vi "Calibration_Load.vi"(11 "Data in":T2={"system"={"info"={"menuSelect"=0, "version"=0, "serial"="Test Sample", "captureActive"=FALSE, "captureBegin"=FALSE, "emptyAndRefill"=FALSE}, "userInfo"={"operatorName"="", "date"=timestamp(2713993200 s since 1904-01-01)}, "camera"={"exposureTime"=0, "aperture"=enum."Item 0", "framerate"=0, "framerateMax"=500, "legacyAttributes"=FALSE}}, "connections"={"arduino"={"connection"="", "status"=FALSE, "openState"=FALSE, "emptyStart"=0}, "pump"={"connection"="MRJ", "status"=FALSE, "command"="", "dispenseSpeed"=100, "flushSize"=100}, "camera"={"cam1"={"connection"="", "status"=FALSE}, "cam2"={"connection"="", "status"=FALSE}}}, "queue"={"process"={"cam1"=refnum, "cam2"=refnum, "queueSize"=0}, "save"={"cam1"=refnum, "cam2"=refnum, "queueSize"=0}, "overloadThreshold"=0}, "imageProcess"={"cam1"={"preAllocation"={"image"="Station", "originalDisplay"="Station", "originalRgb"="Station", "binary"="Station", "save"="Station", "calibrationFull"=refnum, "calibrationDetect"=refnum}, "calibration"={"pathFull"=path "C:/Users/au540322/Desktop/IHS_Project/images/Debris/Debris_0/Debris_0_2019_06_01-23-32-49-686.PNG", "pathDetect"=path "C:/Users/au540322/Desktop/IHS_Project/images/Debris/Debris_0/Debris_0_2019_06_01-23-32-49-686.PNG", "ROI"={"Left"=0, "Top"=0, "Right"=0, "Bottom"=0, "Rotation"=0.0}}}, "cam2"={"preAllocation"={"image"=refnum, "originalDisplay"=refnum, "originalRgb"=refnum, "binary"=refnum, "save"=refnum, "calibrationFull"=refnum, "calibrationDetect"=refnum}, "calibration"={"pathFull"=path "C:/Users/au540322/Desktop/IHS_Project/images/Debris/Debris_0/Debris_0_2019_06_01-23-32-49-686.PNG", "pathDetect"=path "C:/Users/au540322/Desktop/IHS_Project/images/Debris/Debris_0/Debris_0_2019_06_01-23-32-49-686.PNG", "ROI"={"Left"=0, "Top"=0, "Right"=0, "Bottom"=0, "Rotation"=0.0}}}, "process"={"planeExtract"=refnum, "planeSubtract"=refnum, "cropMask"=refnum}, "detection"={"sampleTimeout"=500, "sizeThreshold"=500, "detectionRegionPct"=0.0}}, "sampleData"={"sampleId"="", "projectId"="", "voucherID"="", "speciesName"="", "collectionDate"=timestamp(2713993200 s since 1904-01-01), "sampleStation"="", "location"="", "lat"=0.0, "lon"=0.0, "determiner"="", "sex"="", "otherNotes"=""}, "Session In"=""} {"sampleData"."collectionDate" format="%<%Y-%m-%d>T"; "imageProcess"."detection"."sizeThreshold" min=1; "imageProcess"."cam2"."calibration"."ROI"."Rotation" format="%.2f"; "imageProcess"."cam2"."calibration"."ROI"."Left" scale=0.0..1024.0; "imageProcess"."cam2"."calibration"."ROI"."Right" scale=0.0..1024.0; "imageProcess"."cam1"."calibration"."ROI"."Rotation" format="%.2f"; "imageProcess"."cam1"."calibration"."ROI"."Left" scale=0.0..1024.0; "imageProcess"."cam1"."calibration"."ROI"."Right" scale=0.0..1024.0; "queue"."overloadThreshold" min=1; "queue"."save"."queueSize" min=1; "queue"."process"."queueSize" min=1; "connections"."pump"."flushSize" min=1; "connections"."pump"."dispenseSpeed" min=1; "system"."camera"."framerateMax" min=1; "system"."userInfo"."date" format="%<%Y-%m-%dT%H:%M:%S+%z>T"; "system"."info"."version" items=["Standard", "XL"]; "system"."info"."menuSelect" items=["Session Data", "Extended Setup", "Buffer", "Camera", "Dispenser", "Stats", "Connections"]}) -> (0 "Next State":T1=enum."Wait for Event", 2 "Calibration error?":bool, 3 "Data out":T2={"system"={"info"={"menuSelect"=0, "version"=0, "serial"="Test Sample", "captureActive"=FALSE, "captureBegin"=FALSE, "emptyAndRefill"=FALSE}, "userInfo"={"operatorName"="", "date"=timestamp(2713993200 s since 1904-01-01)}, "camera"={"exposureTime"=0, "aperture"=enum."Item 0", "framerate"=0, "framerateMax"=500, "legacyAttributes"=FALSE}}, "connections"={"arduino"={"connection"="", "status"=FALSE, "openState"=FALSE, "emptyStart"=0}, "pump"={"connection"="", "status"=FALSE, "command"="", "dispenseSpeed"=100, "flushSize"=100}, "camera"={"cam1"={"connection"="", "status"=FALSE}, "cam2"={"connection"="", "status"=FALSE}}}, "queue"={"process"={"cam1"=refnum, "cam2"=refnum, "queueSize"=0}, "save"={"cam1"=refnum, "cam2"=refnum, "queueSize"=0}, "overloadThreshold"=0}, "imageProcess"={"cam1"={"preAllocation"={"image"="Station", "originalDisplay"="Station", "originalRgb"="Station", "binary"="Station", "save"="Station", "calibrationFull"=refnum, "calibrationDetect"=refnum}, "calibration"={"pathFull"=path "C:/Users/au540322/Desktop/IHS_Project/images/Debris/Debris_0/Debris_0_2019_06_01-23-32-49-686.PNG", "pathDetect"=path "C:/Users/au540322/Desktop/IHS_Project/images/Debris/Debris_0/Debris_0_2019_06_01-23-32-49-686.PNG", "ROI"={"Left"=0, "Top"=0, "Right"=0, "Bottom"=0, "Rotation"=0.0}}}, "cam2"={"preAllocation"={"image"=refnum, "originalDisplay"=refnum, "originalRgb"=refnum, "binary"=refnum, "save"=refnum, "calibrationFull"=refnum, "calibrationDetect"=refnum}, "calibration"={"pathFull"=path "C:/Users/au540322/Desktop/IHS_Project/images/Debris/Debris_0/Debris_0_2019_06_01-23-32-49-686.PNG", "pathDetect"=path "C:/Users/au540322/Desktop/IHS_Project/images/Debris/Debris_0/Debris_0_2019_06_01-23-32-49-686.PNG", "ROI"={"Left"=0, "Top"=0, "Right"=0, "Bottom"=0, "Rotation"=0.0}}}, "process"={"planeExtract"=refnum, "planeSubtract"=refnum, "cropMask"=refnum}, "detection"={"sampleTimeout"=500, "sizeThreshold"=500, "detectionRegionPct"=0.0}}, "sampleData"={"sampleId"="", "projectId"="", "voucherID"="", "speciesName"="", "collectionDate"=timestamp(2713993200 s since 1904-01-01), "sampleStation"="", "location"="", "lat"=0.0, "lon"=0.0, "determiner"="", "sex"="", "otherNotes"=""}, "Session In"=""} {"sampleData"."collectionDate" format="%<%Y-%m-%d>T"; "imageProcess"."detection"."sizeThreshold" min=1; "imageProcess"."cam2"."calibration"."ROI"."Rotation" format="%.2f"; "imageProcess"."cam2"."calibration"."ROI"."Left" scale=0.0..1024.0; "imageProcess"."cam2"."calibration"."ROI"."Right" scale=0.0..1024.0; "imageProcess"."cam1"."calibration"."ROI"."Rotation" format="%.2f"; "imageProcess"."cam1"."calibration"."ROI"."Left" scale=0.0..1024.0; "imageProcess"."cam1"."calibration"."ROI"."Right" scale=0.0..1024.0; "queue"."overloadThreshold" min=1; "queue"."save"."queueSize" min=1; "queue"."process"."queueSize" min=1; "connections"."pump"."flushSize" min=1; "connections"."pump"."dispenseSpeed" min=1; "system"."camera"."framerateMax" min=1; "system"."userInfo"."date" format="%<%Y-%m-%dT%H:%M:%S+%z>T"; "system"."info"."version" items=["Standard", "XL"]; "system"."info"."menuSelect" items=["Session Data", "Extended Setup", "Buffer", "Camera", "Dispenser", "Stats", "Connections"]})   [LabVIEW 2022 SP3]
uses:
  controls/Data.ctl
  <vilib>/userdefined/High Color/IMAQdx.ctl
  <vilib>/vision/Image Controls.llb/IMAQ Image.ctl
  controls/State.ctl
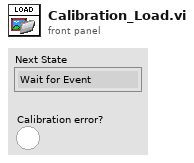
[diagram p1: front panel]
types:
  T1 = typedef "State.ctl" = enum16{"Initialize", "Wait for Event", "Position", "Valve Signal", "Extra Flush", "Valve Cycle", "Valve Open", "Valve Close", "Pump Command", "Pump Cycle", "Empty System", "Start System", "Connect Systems", "Start Image Capture", "Stop Image Capture", "Calibration Pictures", "Close and Refill", "Empty and Refill", "Change Light Intensity", "Reconnect", "CursorIdle", "Exit"}
  T2 = typedef "Data.ctl" = cluster{"system":cluster{"info":cluster{"menuSelect":u16, "version":u16, "serial":string, "captureActive":bool, "captureBegin":bool, "emptyAndRefill":bool}, "userInfo":cluster{"operatorName":string, "date":timestamp}, "camera":cluster{"exposureTime":i32, "aperture":enum32{"Item 0", "Item 1", "Item 2", "Item 3"}, "framerate":i32, "framerateMax":i32, "legacyAttributes":bool}}, "connections":cluster{"arduino":cluster{"connection":refnum<visa-resource-name>, "status":bool, "openState":bool, "emptyStart":u32}, "pump":cluster{"connection":refnum<visa-resource-name>, "status":bool, "command":string, "dispenseSpeed":i32, "flushSize":i32}, "camera":cluster{"cam1":cluster{"connection":T3, "status":bool}, "cam2":cluster{"connection":T3, "status":bool}}}, "queue":cluster{"process":cluster{"cam1":refnum<queue>, "cam2":refnum<queue>, "queueSize":i32}, "save":cluster{"cam1":refnum<queue>, "cam2":refnum<queue>, "queueSize":i32}, "overloadThreshold":i32}, "imageProcess":cluster{"cam1":cluster{"preAllocation":cluster{"image":T4, "originalDisplay":T4, "originalRgb":T4, "binary":T4, "save":T4, "calibrationFull":T4, "calibrationDetect":T4}, "calibration":cluster{"pathFull":path, "pathDetect":path, "ROI":T5}}, "cam2":cluster{"preAllocation":cluster{"image":T4, "originalDisplay":T4, "originalRgb":T4, "binary":T4, "save":T4, "calibrationFull":T4, "calibrationDetect":T4}, "calibration":cluster{"pathFull":path, "pathDetect":path, "ROI":T5}}, "process":cluster{"planeExtract":T4, "planeSubtract":T4, "cropMask":T4}, "detection":cluster{"sampleTimeout":i32, "sizeThreshold":i32, "detectionRegionPct":dbl}}, "sampleData":cluster{"sampleId":string, "projectId":string, "voucherID":string, "speciesName":string, "collectionDate":timestamp, "sampleStation":string, "location":string, "lat":dbl, "lon":dbl, "determiner":string, "sex":string, "otherNotes":string}, "Session In":T3}
  T3 = typedef "IMAQdx.ctl" = refnum<k21>
  T4 = typedef "IMAQ Image.ctl" = refnum<image>
  T5 = typedef "IMAQ Rectangle" = cluster{"Left":i32, "Top":i32, "Right":i32, "Bottom":i32, "Rotation":dbl}
  T6 = typedef "Image Type" = u32
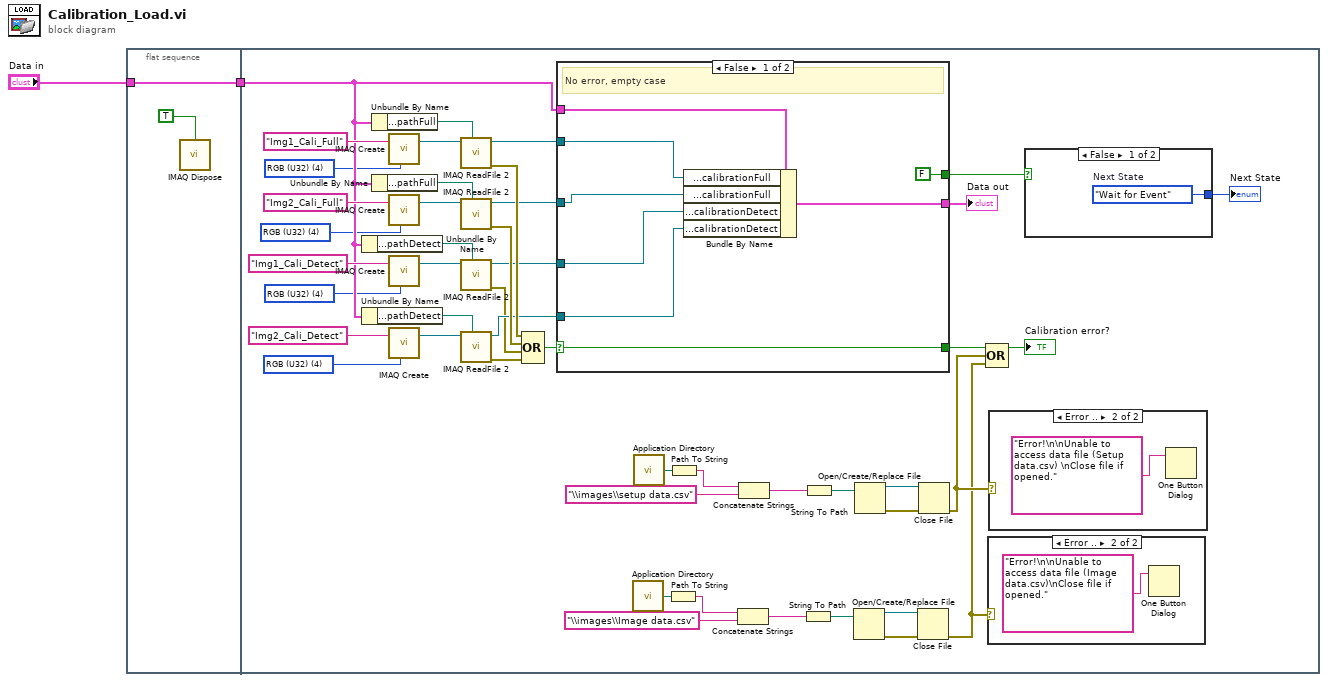
[diagram p0: block diagram]
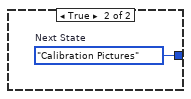
[diagram p4: hidden frame]
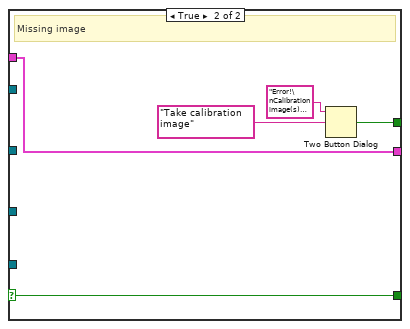
[diagram p5: hidden frame]
diagram:
  n1 = flat-sequence {
    tunnel: "Data in" -> [w4]
    tunnel: [w4] -> w1
    tunnel: w1 -> [w28]
    frame #0 {
      n2 = call "IMAQ Dispose"("All Images? (No)"=TRUE) -> ()  [unwired: 5 in, 1 out]
    }
    frame #1 {
      w16 = T6 4 items=["Grayscale (U8)", "Grayscale (I16)", "Grayscale (SGL)", "Complex (CSG)", "RGB (U32)", "HSL (U32)", "RGB (U64)", "Grayscale (U16)"] ("Image Type")
      w17 = T6 4 items=["Grayscale (U8)", "Grayscale (I16)", "Grayscale (SGL)", "Complex (CSG)", "RGB (U32)", "HSL (U32)", "RGB (U64)", "Grayscale (U16)"] ("Image Type")
      w18 = T6 4 items=["Grayscale (U8)", "Grayscale (I16)", "Grayscale (SGL)", "Complex (CSG)", "RGB (U32)", "HSL (U32)", "RGB (U64)", "Grayscale (U16)"] ("Image Type")
      w19 = T6 4 items=["Grayscale (U8)", "Grayscale (I16)", "Grayscale (SGL)", "Complex (CSG)", "RGB (U32)", "HSL (U32)", "RGB (U64)", "Grayscale (U16)"] ("Image Type")
      n3 = Unbundle By Name(w28) -> ("imageProcess.cam1.calibration.pathDetect"=w29:path)
      n4 = Unbundle By Name(w28) -> ("imageProcess.cam2.calibration.pathDetect"=w27:path)
      n5 = Unbundle By Name(w28) -> ("imageProcess.cam1.calibration.pathFull"=w49:path)
      n6 = Unbundle By Name(w28) -> ("imageProcess.cam2.calibration.pathFull"=w46:path)
      n7 = call "IMAQ Create"("Image Name"="Img1_Cali_Full", "Image Type"=w19) -> ("New Image"=w50:T4)  [unwired: 2 in, 2 out]
      n8 = call "IMAQ Create"("Image Name"="Img2_Cali_Full", "Image Type"=w16) -> ("New Image"=w47:T4)  [unwired: 2 in, 2 out]
      n9 = call "IMAQ Create"("Image Name"="Img1_Cali_Detect", "Image Type"=w18) -> ("New Image"=w35:T4)  [unwired: 2 in, 2 out]
      n10 = call "IMAQ Create"("Image Name"="Img2_Cali_Detect", "Image Type"=w17) -> ("New Image"=w33:T4)  [unwired: 2 in, 2 out]
      n11 = call "IMAQ ReadFile 2"("File Path"=w49, "Image"=w50) -> ("error out"=w43:errorcluster, "Image Out"=w38:T4)  [unwired: 5 in, 3 out]
      n12 = call "IMAQ ReadFile 2"("File Path"=w46, "Image"=w47) -> ("error out"=w44:errorcluster, "Image Out"=w39:T4)  [unwired: 5 in, 3 out]
      n13 = call "IMAQ ReadFile 2"("File Path"=w29, "Image"=w35) -> ("error out"=w31:errorcluster, "Image Out"=w34:T4)  [unwired: 5 in, 3 out]
      n14 = call "IMAQ ReadFile 2"("File Path"=w27, "Image"=w33) -> ("error out"=w30:errorcluster, "Image Out"=w32:T4)  [unwired: 5 in, 3 out]
      n15 = Compound Arithmetic op=OR(w43, w44, w31, w30) -> (w45:bool)
      n16 = case shown="False" w45 {
        selector: w45 -> [w60 w64]
        tunnel: w28 -> [w63 w66]
        tunnel: [w62 w66] -> w42
        tunnel: [FALSE ("T button?") w65] -> w41
        tunnel: [w60 w64] -> w8
        tunnel: w39 -> [w59 _]
        tunnel: w38 -> [w58 _]
        tunnel: w34 -> [w57 _]
        tunnel: w32 -> [w56 _]
        frame False {
          # "No error, empty case"
          n17 = Bundle By Name(cluster=w63, "imageProcess.cam1.preAllocation.calibrationFull"=w58, "imageProcess.cam2.preAllocation.calibrationFull"=w59, "imageProcess.cam1.preAllocation.calibrationDetect"=w57, "imageProcess.cam2.preAllocation.calibrationDetect"=w56) -> (w62:T2)
        }
        frame True {
          # "Missing image"
          n18 = Two Button Dialog(message="Error!\nCalibration image(s) missing!", 2:"Take calibration image" ("T button name (\"OK\")")) -> (T button?=w65:bool)  [unwired: 1 in]
        }
      }
      "Data out" <- w42
      n19 = call <vilib>:"Application Directory.vi"() -> ("Application Directory"=w15:path)
      n20 = call <vilib>:"Application Directory.vi"() -> ("Application Directory"=w26:path)
      n21 = Path To String(path=w15) -> (string=w14:string)
      n22 = Path To String(path=w26) -> (string=w25:string)
      n23 = Concatenate Strings(w14, "\\images\\Image data.csv") -> (w12:string)
      n24 = Concatenate Strings(w25, "\\images\\setup data.csv") -> (w23:string)
      n25 = String To Path(string=w12) -> (path=w11:path)
      n26 = String To Path(string=w23) -> (path=w22:path)
      n27 = Open/Create/Replace File(file path (use dialog)=w11) -> (refnum out=w10:refnum<file>, error out=w9:errorcluster)  [unwired: 5 in, 1 out]
      n28 = Open/Create/Replace File(file path (use dialog)=w22) -> (refnum out=w21:refnum<file>, error out=w20:errorcluster)  [unwired: 5 in, 1 out]
      n29 = Close File(refnum=w10, error in=w9) -> (error out=w5:errorcluster)  [unwired: 1 out]
      n30 = Close File(refnum=w21, error in=w20) -> (error out=w7:errorcluster)  [unwired: 1 out]
      n31 = Compound Arithmetic op=OR(w8, w7, w5) -> (→"Calibration error?":bool)
      n32 = case shown="Error .." w5 {
        frame No Error {
        }
        frame Error {
          n33 = One Button Dialog(message="Error!\n\nUnable to access data file (Image data.csv)\nClose file if opened.") -> ()  [unwired: 1 in, 1 out]
        }
      }
      n34 = case shown="Error .." w7 {
        frame No Error {
        }
        frame Error {
          n35 = One Button Dialog(message="Error!\n\nUnable to access data file (Setup data.csv) \nClose file if opened.") -> ()  [unwired: 1 in, 1 out]
        }
      }
      n36 = case shown="False" w41 {
        tunnel: [w54 w55] -> w40
        frame False {
          w54 = State."Wait for Event"  # Next State
        }
        frame True {
          w55 = State."Calibration Pictures"  # Next State
        }
      }
      "Next State" <- w40
    }
  }
